vi "test_mean_map.vi"() -> ()   [LabVIEW 2009]
doc: "Copyright (C) 2009, Stepan A. Baranov\nweb: http://www.OCTLab.org/\nemail: stepan@baranov.su"
uses:
  OCTLib.dll
panel:
  out "error out":errorcluster
  out "radius":i32
  out "width":i32
  out "height":i32
  in  "Small/Big":bool
  out "loop #":i32
  out "RSM_STAT time":u32
  out "LabView time":u32
  out "RSM_STAT Array":dbl[][](array[numeric])
  out "LabView Array":dbl[][](array[numeric])
  in  "stop":bool
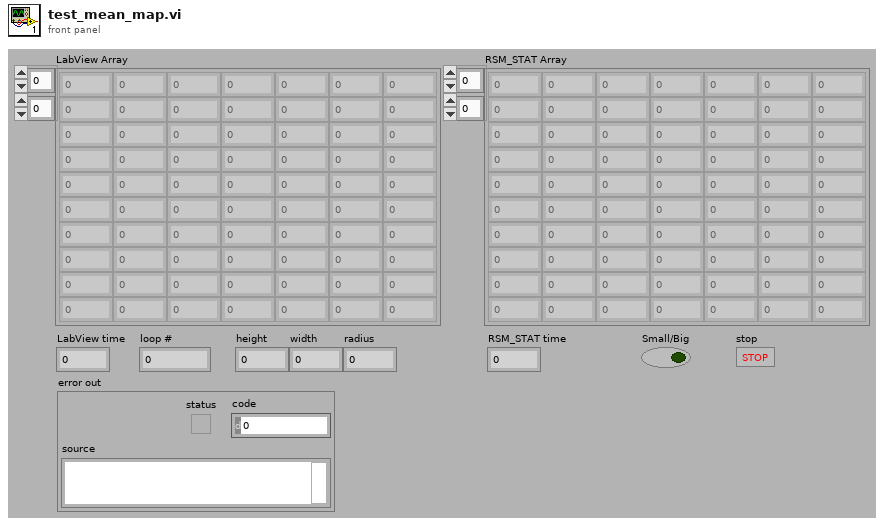
[diagram p1: front panel]
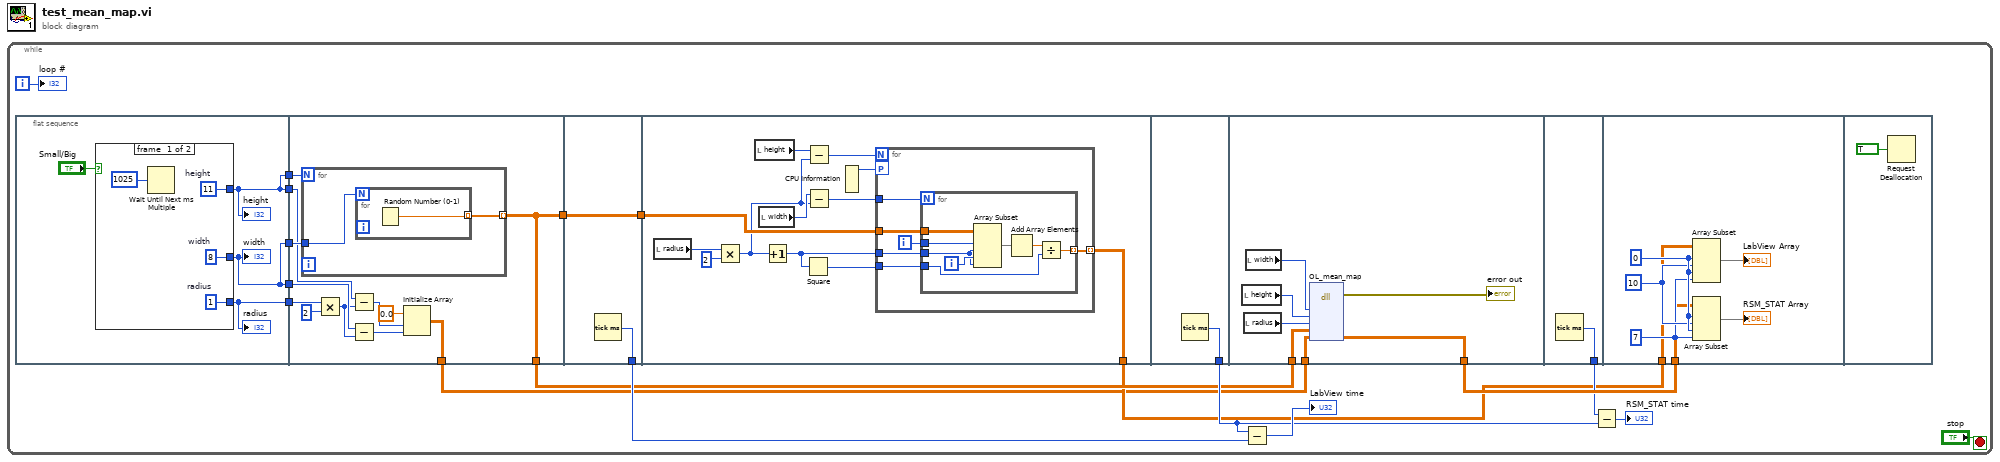
[diagram p0: block diagram]
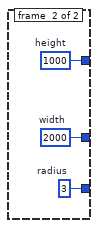
[diagram p2: hidden frame]
diagram:
  n1 = while {
    i -> [w11]
    stop <- "stop" stop-if-true
    n2 = flat-sequence {
      tunnel: [w19] -> w7
      tunnel: [w20] -> w6
      tunnel: [w21] -> w4
      tunnel: [w20] -> w3
      tunnel: [w19] -> w2
      tunnel: [w39] -> w10
      tunnel: [w39] -> w8
      tunnel: w7 -> [w41]
      tunnel: w6 -> [w40]
      tunnel: w4 -> [w37]
      tunnel: w3 -> [w35]
      tunnel: w2 -> [w33]
      tunnel: [w30] -> w1
      tunnel: [w46] -> w16
      tunnel: [w45] -> w9
      tunnel: w8 -> [w45]
      tunnel: w9 -> [w58]
      tunnel: [w54] -> w5
      tunnel: [w73] -> w13
      tunnel: w10 -> [w79]
      tunnel: [w78] -> w17
      tunnel: w1 -> [w80]
      tunnel: [w81] -> w14
      tunnel: w17 -> [w84]
      tunnel: w5 -> [w83]
      frame #0 {
        n3 = case shown="True" "Small/Big" {
          tunnel: [w24 w29] -> w20
          tunnel: [w25 w28] -> w19
          tunnel: [w26 w27] -> w21
          frame #0 {
            w26 = 1  # radius
            w25 = 8  # width
            w24 = 11  # height
            n4 = Wait Until Next ms Multiple(millisecond multiple=u32 1025) -> ()  [unwired: 1 out]
          }
          frame #1 {
            w27 = 3  # radius
            w28 = 2000  # width
            w29 = 1000  # height
          }
        }
        "height" <- w20
        "width" <- w19
        "radius" <- w21
      }
      frame #1 {
        n5 = for {
          N: w40 -> [_]
          tunnel: w41 -> [w43]
          tunnel: [w42] -> w39 mode=indexing
          n6 = for {
            N: w43 -> [_]
            tunnel: [w44] -> w42 mode=indexing
            n7 = Random Number (0-1)() -> (number: 0 to 1=w44:dbl)
          }
        }
        n8 = Multiply(x=w37, y=2) -> (x*y=w32:i32)
        n9 = Subtract(x=w35, y=w32) -> (x-y=w34:i32)
        n10 = Subtract(x=w33, y=w32) -> (x-y=w31:i32)
        n11 = Initialize Array(0.0 ("element"), w34, w31) -> (w30:dbl[][])
      }
      frame #2 {
        n12 = Tick Count (ms)() -> (millisecond timer value=w46:u32)
      }
      frame #3 {
        n13 = local read "radius"() -> (w57:i32)
        n14 = Multiply(x=w57, y=2) -> (x*y=w49:i32)
        n15 = local read "height"() -> (w52:i32)
        n16 = local read "width"() -> (w50:i32)
        n17 = Increment(x=w49) -> (x+1=w53:i32)
        n18 = Square(x=w53) -> (x^2=w55:i32)
        n19 = Subtract(x=w52, y=w49) -> (x-y=w51:i32)
        n20 = Subtract(x=w50, y=w49) -> (x-y=w48:i32)
        n21 = CPU Information() -> (4:w47:i32)  [unwired: 3 out]
        n22 = for {
          N: w51 -> [_]
          tunnel: w58 -> [w63]
          tunnel: w55 -> [w62]
          tunnel: [w61] -> w54 mode=indexing
          tunnel: w53 -> [w60]
          tunnel: w48 -> [w59]
          workers-P: w47 -> [_]
          i -> [w64]
          n23 = for {
            N: w59 -> [_]
            tunnel: w64 -> [w71]
            tunnel: w63 -> [w69]
            tunnel: w62 -> [w68]
            tunnel: [w66] -> w61 mode=indexing
            tunnel: w60 -> [w65]
            i -> [w70]
            n24 = Array Subset(array=w69, index (row)=w71, length (row)=w65, index (col)=w70, length (col)=w65) -> (w67:dbl[][])
            n25 = Add Array Elements(numeric array=w67) -> (sum=w72:dbl)
            n26 = Divide(x=w72, y=w68) -> (x/y=w66:dbl)
          }
        }
      }
      frame #4 {
        n27 = Tick Count (ms)() -> (millisecond timer value=w73:u32)
      }
      frame #5 {
        n28 = local read "height"() -> (w76:i32)
        n29 = local read "radius"() -> (w75:i32)
        n30 = local read "width"() -> (w77:i32)
        n31 = dll-call lib="OCTLib.dll" fn="OL_mean_map"("width"=w77, "height"=w76, "radius"=w75, "input"=w79, "output"=w80) -> (error out=→"error out":errorcluster, "output"=w78:dbl[][])  [unwired: 8 in, 1 out]
      }
      frame #6 {
        n32 = Tick Count (ms)() -> (millisecond timer value=w81:u32)
      }
      frame #7 {
        w87 = 10 ("length")
        w86 = 7 ("length")
        w88 = 0 ("index")
        n33 = Array Subset(array=w83, index (row)=w88, length (row)=w87, index (col)=w88, length (col)=w86) -> (→"LabView Array":dbl[][])
        n34 = Array Subset(array=w84, index (row)=w88, length (row)=w87, index (col)=w88, length (col)=w86) -> (→"RSM_STAT Array":dbl[][])
      }
      frame #8 {
        n35 = Request Deallocation(TRUE ("flag")) -> ()
      }
    }
    n36 = Subtract(x=w13, y=w16) -> (x-y=→"LabView time":u32)
    n37 = Subtract(x=w14, y=w13) -> (x-y=→"RSM_STAT time":u32)
    "loop #" <- w11
  }
